vi "Start Sending.vi"(7 "Response":refnum<class>, 10 "error in (no error)":errorcluster, 11 "RequestTraceLog in":refnum<class "RequestTraceLog.lvclass">) -> (2 "error out":errorcluster, 3 "RequestTraceLog out":refnum<class "RequestTraceLog.lvclass">)   [LabVIEW 2020, in "HTTP Server.lvlib" / "RequestTraceLog.lvclass"]
uses:
  RequestTraceLog.lvclass
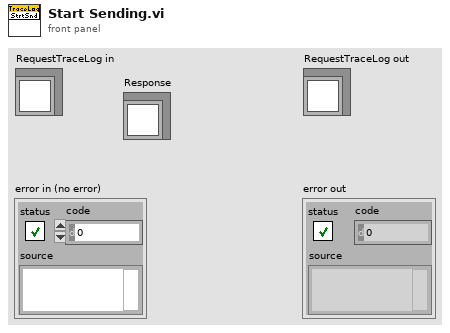
[diagram p1: front panel]
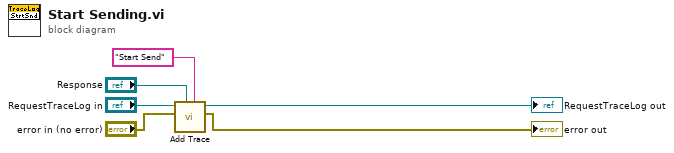
[diagram p0: block diagram]
diagram:
  n1 = call "Add Trace.vi"("Info"="Start Send", "LabVIEW Object"="Response", "error in (no error)"="error in (no error)", "RequestTraceLog in"="RequestTraceLog in") -> ("error out"=→"error out":errorcluster, "RequestTraceLog out"=→"RequestTraceLog out":refnum<class "RequestTraceLog.lvclass">)  [unwired: 6 in]
